vi "manifold config error box update (sub-vi).vi"(8 "error in (no error)":errorcluster, 10 "manifold config error array":bool[][](array[boolean]), 11 "manifold config array refnum":refnum<vi>) -> (0 "error out":errorcluster, 3 "manifold config array refnum out":refnum<vi>)   [LabVIEW 2021]
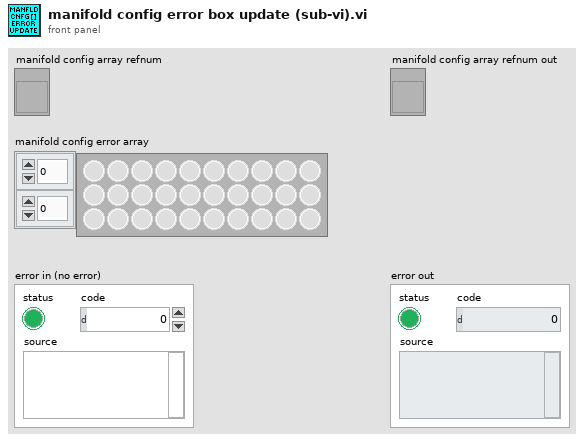
[diagram p1: front panel]
types:
  T1 = typedef "stimulator configuration cluster (type def).ctl" = cluster{"position:":T2, "port connections:":T3[]}
  T2 = typedef "stimulator selection.ctl" = enum16{"left", "middle", "right"}
  T3 = typedef "single port single odor cluster.ctl" = cluster{"port number":T4, "connected odor":T5, "error":bool, "odor color":T6}
  T4 = typedef "port number (type def).ctl" = enum16{"port 1", "port 2", "port 3", "port 4", "port 5", "port 6", "port 7", "port 8"}
  T5 = typedef "odor selection (type def).ctl" = enum16{"[none]", "odor 1", "odor 2", "odor 3", "odor 4", "odor 5", "odor 6", "odor 7", "odor 8", "odor 9", "odor 10"}
  T6 = typedef "odor color (type def).ctl" = u16
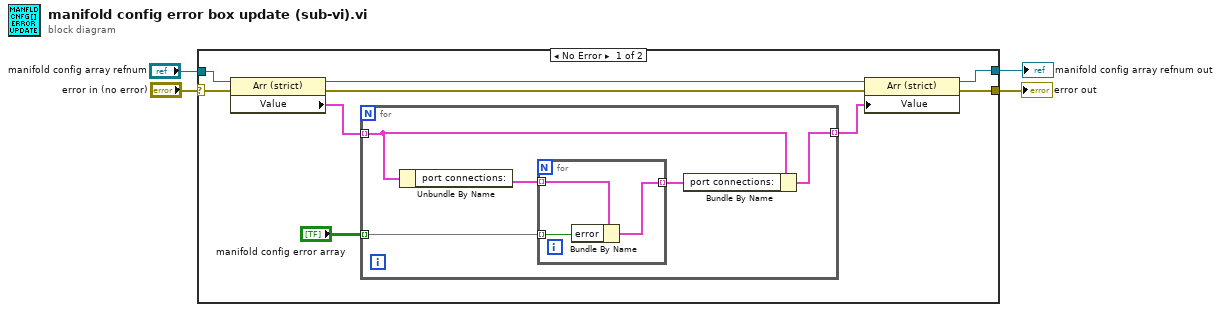
[diagram p0: block diagram]
diagram:
  n1 = case shown="No Error" "error in (no error)" {
    selector: "error in (no error)" -> [w11 w22]
    tunnel: [w13 w22] -> w4
    tunnel: [w7 w23] -> w2
    tunnel: "manifold config array refnum" -> [w6 w23]
    frame No Error {
      n2 = property class="Arr (strict)"(reference=w6, error in=w11) -> (reference out=w8:refnum<vi>, error out=w12:errorcluster, "Value"=w9:T1[])
      n3 = for {
        tunnel: w9 -> [w17] mode=indexing
        tunnel: [w15] -> w10 mode=indexing
        tunnel: "manifold config error array" -> [w14] mode=indexing
        n4 = Unbundle By Name(w17) -> ("port connections:"=w18:T3[])
        n5 = for {
          tunnel: w18 -> [w21] mode=indexing
          tunnel: [w20] -> w16 mode=indexing
          tunnel: w14 -> [w19] mode=indexing
          n6 = Bundle By Name(cluster=w21, "error"=w19) -> (w20:T3)
        }
        n7 = Bundle By Name(cluster=w17, "port connections:"=w16) -> (w15:T1)
      }
      n8 = property class="Arr (strict)"(reference=w8, error in=w12, "Value"=w10) -> (reference out=w7:refnum<vi>, error out=w13:errorcluster)
    }
    frame Error {
    }
  }
  "error out" <- w4
  "manifold config array refnum out" <- w2
